vi "Create.vi"(6 "Year of license":i32, 8 "error in (no error)":errorcluster, 10 "Company_Info":T1, 11 "Software License Manager in":refnum<class "Software License Manager.lvclass">) -> (0 "error out":errorcluster, 1 "ok?":bool, 3 "Software License Manager out":refnum<class "Software License Manager.lvclass">)   [LabVIEW 2021, in "Software License Manager.lvclass"]
uses:
  Software License Manager.lvclass
  Software License Manager.lvclass/Software License Manager.ctl
  Board/Board.lvclass/Board.ctl
  Board/Read Product ID.vi
  <vilib>/httpClient/POSTBuffer.vi
  <vilib>/httpClient/LabVIEWHTTPClient.lvlib
  Board/Board.lvclass
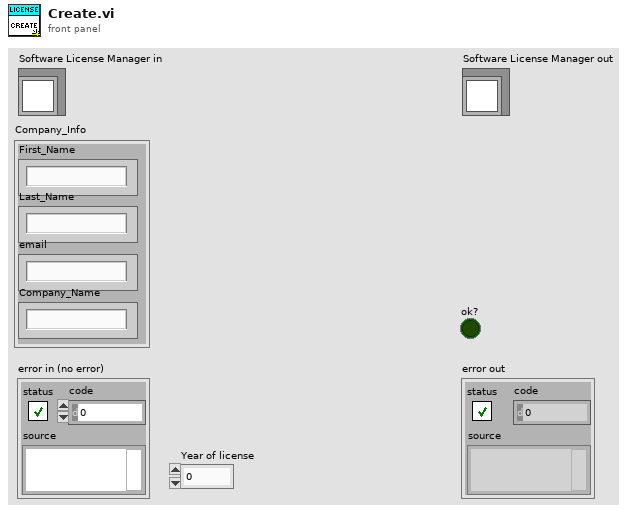
[diagram p1: front panel]
types:
  T1 = cluster{"First_Name":string, "Last_Name":string, "email":string, "Company_Name":string}
  T2 = typedef "LVDateTimeRec.ctl" = cluster{"fractional second":dbl, "second":i32, "minute":i32, "hour":i32, "day of month":i32, "month":i32, "year":i32, "day of week":i32, "day of year":i32, "DST":i32}
  T3 = typedef "LabVIEWHTTPClient.lvlib/ClientHandle.ctl" = refnum<k1>
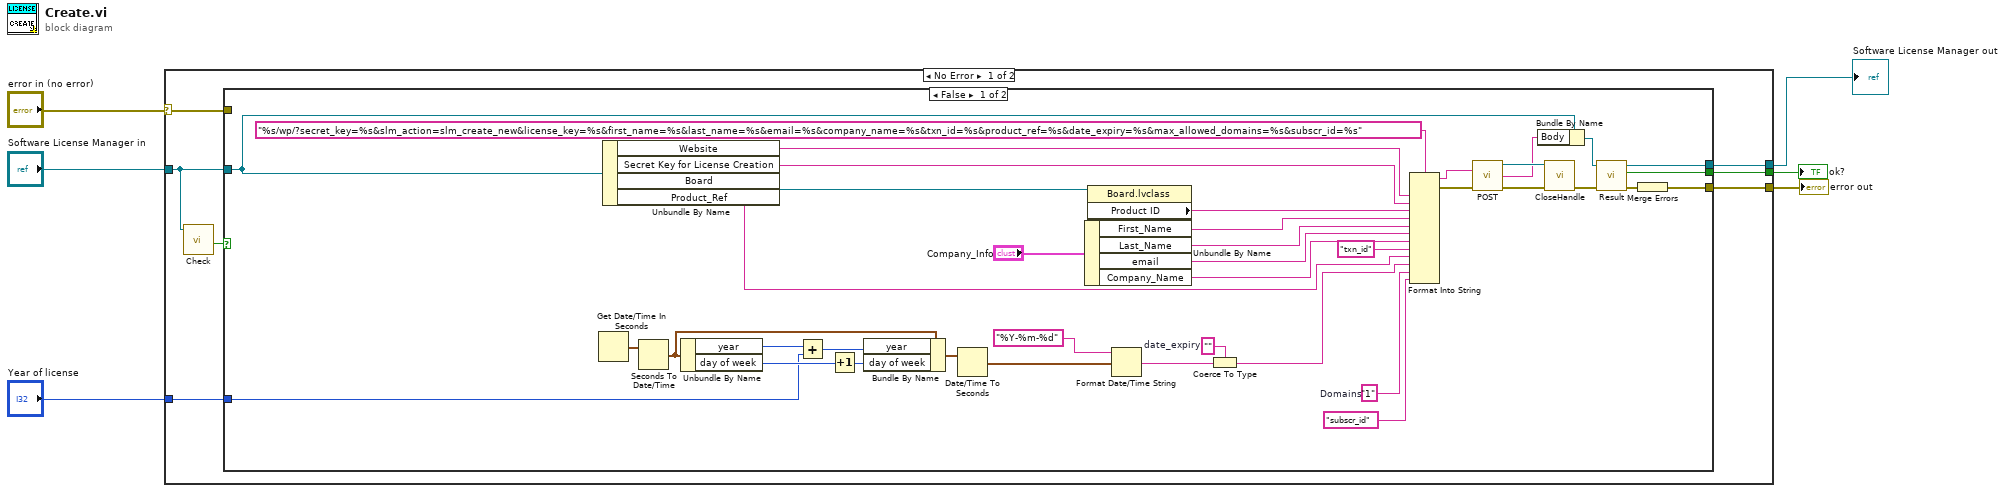
[diagram p0: block diagram]
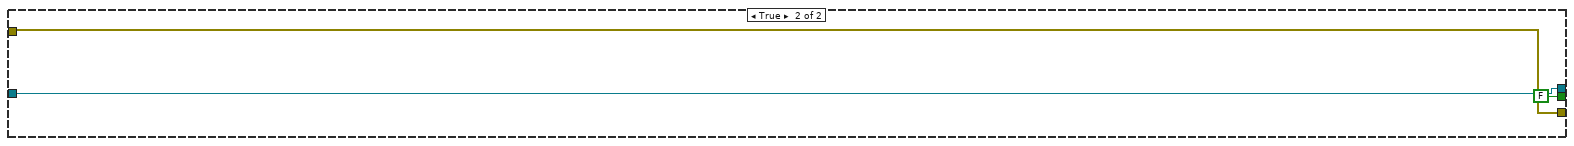
[diagram p2: hidden frame]
diagram:
  n1 = case shown="No Error" "error in (no error)" {
    selector: "error in (no error)" -> [w13 w57]
    tunnel: [w12 w57] -> w5
    tunnel: [w11 w56] -> w3
    tunnel: "Software License Manager in" -> [w9 w56]
    tunnel: [w10 _] -> w2
    tunnel: "Year of license" -> [w7 _]
    frame No Error {
      n2 = call-dynamic "Check.vi"("Software License Manager in"=w9) -> ("ok?"=w8:bool)  [unwired: 7 in, 3 out]
      n3 = case shown="False" w8 {
        tunnel: w13 -> [_ w55]
        tunnel: [w40 w55] -> w12
        tunnel: [w36 w54] -> w11
        tunnel: [w35 FALSE ("ok?")] -> w10
        tunnel: w9 -> [w34 w54]
        tunnel: w7 -> [w16 _]
        frame False {
          w31 = ""  # date_expiry
          w22 = "1"  # Domains
          n4 = Get Date/Time In Seconds() -> (seconds since 1Jan1904=w24:timestamp)
          n5 = Unbundle By Name(w34) -> ("Website"=w51:string, "Secret Key for License Creation"=w14:string, "Board"=w20:refnum<class "Board.lvclass">, "Product_Ref"=w15:string)
          n6 = Seconds To Date/Time(time stamp (now)=w24) -> (date time rec=w27:T2)  [unwired: 1 in]
          n7 = Unbundle By Name(w27) -> ("year"=w18:i32, "day of week"=w25:i32)
          n8 = Add(x=w18, y=w16) -> (x+y=w17:i32)
          n9 = Increment(x=w25) -> (x+1=w26:i32)
          n10 = Bundle By Name(cluster=w27, "year"=w17, "day of week"=w26) -> (w28:T2)
          n11 = Date/Time To Seconds(2:w28) -> (0:w29:timestamp)  [unwired: 1 in]
          n12 = Unbundle By Name("Company_Info") -> ("First_Name"=w49:string, "Last_Name"=w48:string, "email"=w47:string, "Company_Name"=w46:string)
          n13 = property class="Board.lvclass"(reference=w20) -> ("Product ID"=w19:string)  [unwired: 1 in, 2 out]
          n14 = Format Date/Time String(time format string (%c)="%Y-%m-%d", seconds (now)=w29) -> (date/time string=w30:string)  [unwired: 1 in]
          n15 = Coerce To Type(0:w30, 1:w31) -> (2:w23:string)
          n16 = Format Into String(format string="%s/wp/?secret_key=%s&slm_action=slm_create_new&license_key=%s&first_name=%s&last_name=%s&email=%s&company_name=%s&txn_id=%s&product_ref=%s&date_expiry=%s&max_allowed_domains=%s&subscr_id=%s", w51, w14, w19, w49, w48, w47, w46, "txn_id", w15, w23, w22, "subscr_id") -> (resulting string=w45:string, error out=w44:errorcluster)  [unwired: 2 in]
          n17 = call-poly <vilib>:"POST.vi"("url"=w45, "error in (no error)"=w44) -> ("client handle out"=w42:T3, "body"=w38:string, "error out"=w43:errorcluster)  [unwired: 10 in, 1 out]
          n18 = Bundle By Name(cluster=w34, "Body"=w38) -> (w37:refnum<class "Software License Manager.lvclass">)
          n19 = call <vilib>:"CloseHandle.vi"("client handle"=w42, "error in (no error)"=w43) -> ("error out"=w41:errorcluster)  [unwired: 13 in]
          n20 = call-dynamic "Result.vi"("error in (no error)"=w41, "Software License Manager in"=w37) -> ("error out"=w39:errorcluster, "ok?"=w35:bool, "Software License Manager out"=w36:refnum<class "Software License Manager.lvclass">)  [unwired: 6 in, 1 out]
          n21 = Merge Errors(w39) -> (w40:errorcluster)
        }
        frame True {
        }
      }
    }
    frame Error {
    }
  }
  "error out" <- w5
  "Software License Manager out" <- w3
  "ok?" <- w2
